vi "XML_method_params.vi"(0 "XML-message":string="<?xml version=\"1.0\"?>\n<methodCall>\n <methodName>jil.runvi</methodName>\n <params>\n   <param>\n     <value><i4>41</i4></value>\n   </param>\n   <param>\n     <value><int>-17</int></value>\n   </param>\n   <param>\n     <value><boolean>1</boolean></value>\n   </param>\n   <param>\n     <value><string>Hola</string></value>\n   </param>\n   <param>\n     <value>esto es un string \"a pelo\"</value>\n   </param>\n   <param>\n     <value><double>-187.217</double></value>\n   </param>\n   <param>\n     <value><dateTime.iso8601>19980717T14:08:55</dateTime.iso8601></value>\n   </param>\n   <param>\n     <value><base64>eW91IGNhbid0IHJlYWQgdGhpcyE=</base64></value>\n   </param>\n\n   <param>\n     <value>\n     <struct>\n       <member>\n            <name>lowerBound</name>\n           <value><i4>18</i4></value>\n       </member>\n        <member>\n           <name>upperBound</name>\n           <value><i4>139</i4></value>\n         </member>\n       </struct>\n      </value>\n   </param>\n\n   <param>\n     <value>\n     <array>\n        <data>\n           <value><i4>12</i4></value>\n           <value><string>Egypt</string></value>\n           <value><boolean>0</boolean></value>\n           <value><i4>-31</i4></value>\n        </data>\n       </array>\n      </value>\n    </param>\n\n </params>\n</methodCall>\n\n" caption="Result") -> (1 "ParsingErrors":string="<?xml version=\"1.0\" encoding=\"UTF-8\"?>\n<methodResponse>\n  <fault>\n    <value>\n      <struct>\n        <member>\n          <name>faultCode</name>\n          <value><int>811</int></value>\n        </member>\n        <member>\n          <name>faultString</name>\n          <value><string>Error in value:\n\" &ampvalue>\n     <value><i4>41</i4></value>\n   </value>\"</string></value>\n        </member>\n     </struct>\n    </value>\n  </fault>\n</methodResponse>", 2 "Values":variant[](array[variant]), 3 "Types":T1(array[ring])=[enum."int"], 4 "Method":T2(ring)=enum."RunVI")   [LabVIEW 2010]
panel:
  out "tag_list":string[](array[string])
  out "body_temp":string="\n\n"
  out "XML ok":bool
  out "RestOfParams":string
  out "XMLparams":string[](array[string])=["\n     <value><i4>41</i4></value>\n   ", "\n     <value><int>-17</int></value>\n   ", "\n     <value><boolean>1</boolean></value>\n   ", "\n     <value><string>Hola</string></value>\n   ", "\n     <value>esto es un string \"a pelo\"</value>\n   ", "\n     <value><double>-187.217</double></value>\n   ", "\n     <value><dateTime.iso8601>19980717T14:08:55</dateTime.iso8601></value>\n   ", "\n     <value><base64>eW91IGNhbid0IHJlYWQgdGhpcyE=</base64></value>\n   ", "\n     <value>\n     <struct>\n       <member>\n            <name>lowerBound</name>\n           <value><i4>18</i4></value>\n       </member>\n        <member>\n           <name>upperBound</name>\n           <value><i4>139</i4></value>\n         </member>\n       </struct>\n      </value>\n   ", "\n     <value>\n     <array>\n        <data>\n           <value><i4>12</i4></value>\n           <value><string>Egypt</string></value>\n           <value><boolean>0</boolean></value>\n           <value><i4>-31</i4></value>\n        </data>\n       </array>\n      </value>\n    "]
  out "header":string="<?xml version=\"1.0\"?>"
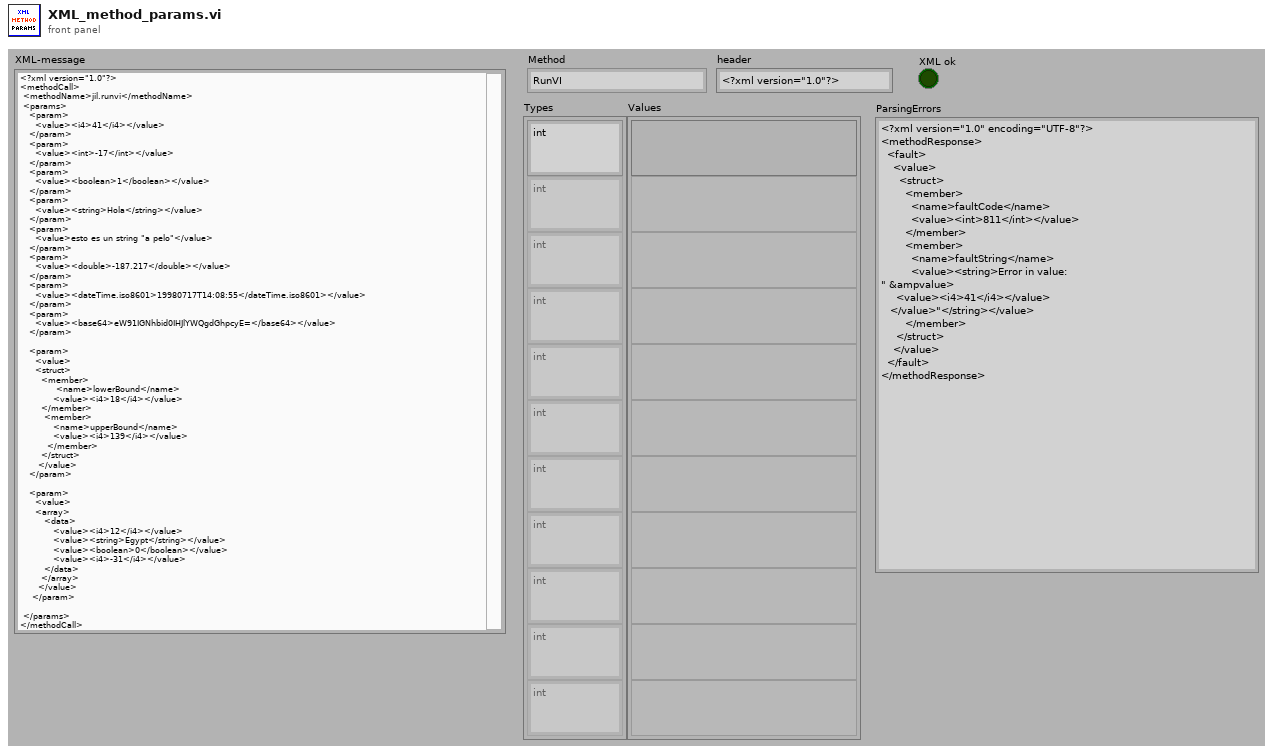
[diagram p1: front panel]
types:
  T1 = enum16{"int", "boolean", "string", "double", "dateTime", "base64", "struct", "array"}[]
  T2 = enum16{"Connect", "Authenticate", "OpenVI", "RunVI", "SyncVI", "StopVI", "CloseVI", "Disconnect"}
  T3 = enum16{"int", "boolean", "string", "double", "dateTime", "base64", "struct", "array"}
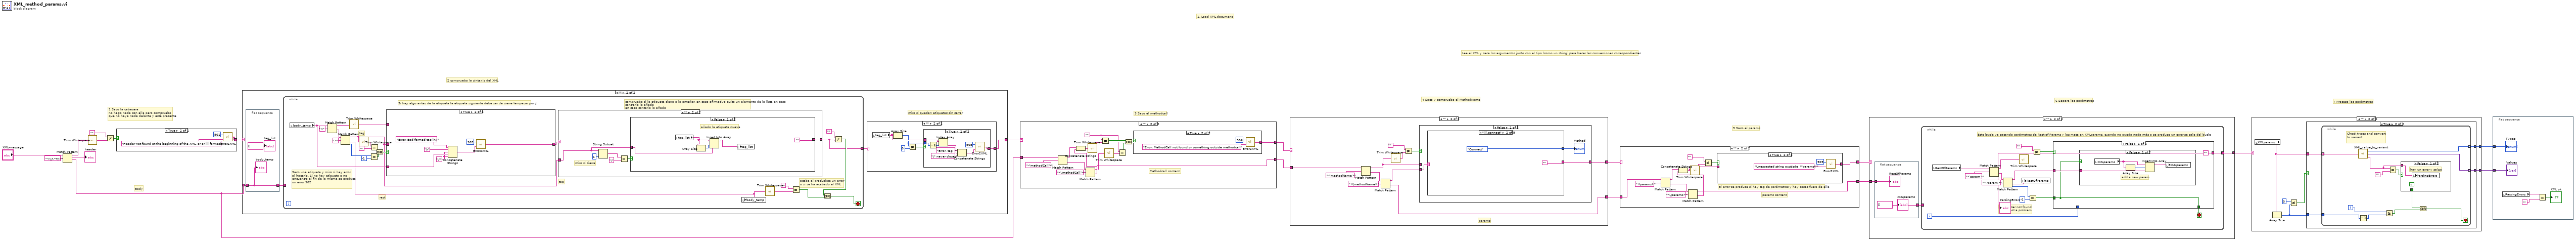
[diagram p0: block diagram]
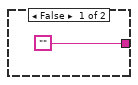
[diagram p2: hidden frame]
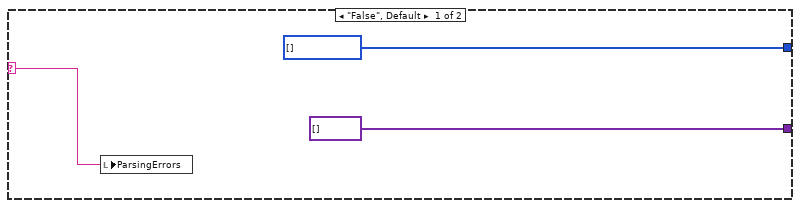
[diagram p3: hidden frame]
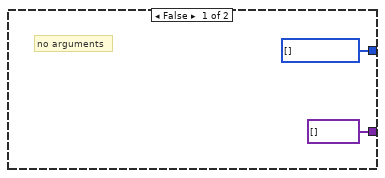
[diagram p4: hidden frame]
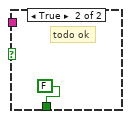
[diagram p5: hidden frame]
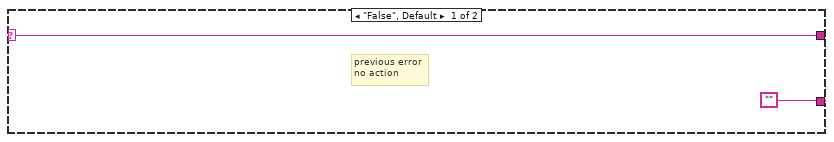
[diagram p6: hidden frame]
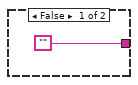
[diagram p7: hidden frame]
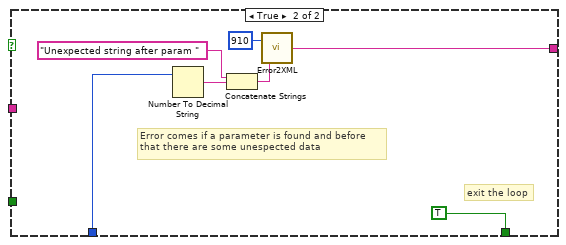
[diagram p10: hidden frame]
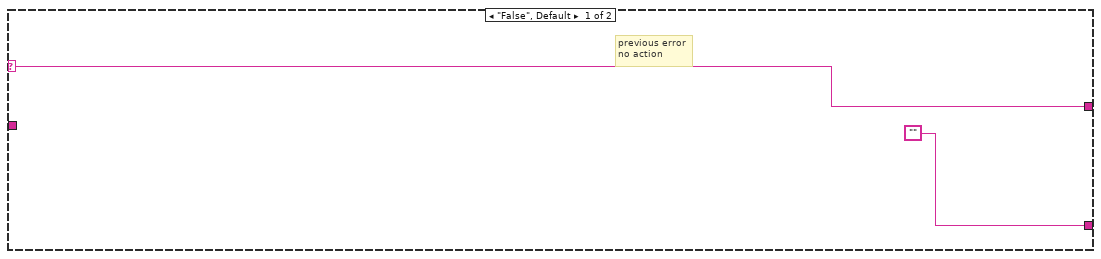
[diagram p11: hidden frame]
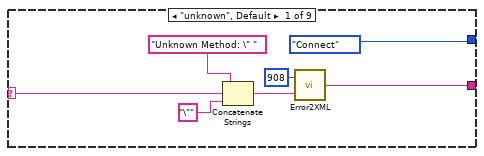
[diagram p12: hidden frame]
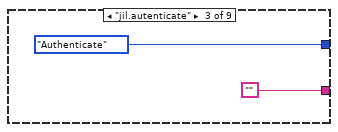
[diagram p13: hidden frame]
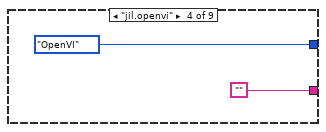
[diagram p14: hidden frame]
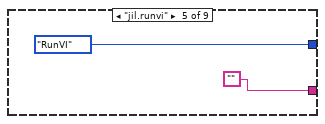
[diagram p15: hidden frame]
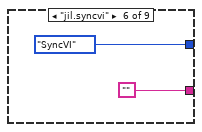
[diagram p16: hidden frame]
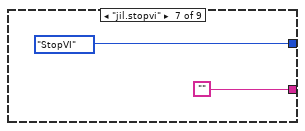
[diagram p17: hidden frame]
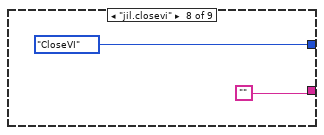
[diagram p18: hidden frame]
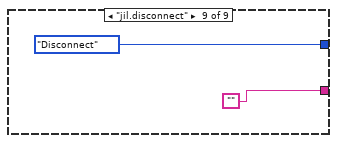
[diagram p19: hidden frame]
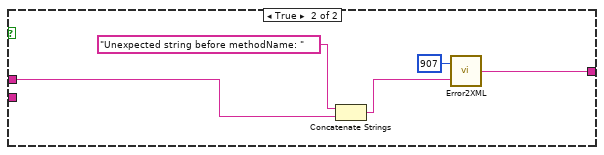
[diagram p20: hidden frame]
diagram:
  # "7 Proceso los parámetros"
  # "6 Separa los parámetros"
  # "5 Saco el params"
  # "4 Saco y compruebo el MethodName"
  # "3 Saco el methodcall"
  # "1 Saco la cabecera\nno hago nada con ella pero compruebo \nque no haya nada delante y esté presente"
  # "Body"
  # "2 compruebo la sintaxis del XML"
  # "1. Load XML document"
  # "Lee el XML y saca los argumentos junto con el tipo (como un string) para hacer las conversiones correspondientes"
  n1 = Match Pattern(string="XML-message", regular expression="<\\?.*?\\>") -> (before substring=w8:string, match substring=→"header":string, after substring=w2:string)  [unwired: 1 in, 1 out]
  n2 = call <vilib>:"Trim Whitespace.vi"("string"=w8) -> ("trimmed string"=w9:string)  [unwired: 1 in]
  n3 = Not Equal?(x="", y=w9) -> (x != y?=w5:bool)
  n4 = case shown="True" w5 {
    tunnel: ["" w21] -> w3
    frame False {
    }
    frame True {
      n5 = call "Error2XML.vi"("FailDescriptor"="Header not found at the beginning of the XML, or or ill formed ", "FailID"=901) -> ("ErrorXML"=w21:string)
    }
  }
  n6 = case shown="\"\"" w3 {
    selector: w3 -> [w24 _]
    tunnel: [w24 w25] -> w19
    tunnel: w2 -> [_ w28]
    frame "False", Default {
      # "previous error\nno action"
    }
    frame "" {
      # "miro si quedan etiquetas sin cerrar"
      n7 = flat-sequence {
        tunnel: [w46] -> w27
        tunnel: w28 -> [w46]
        frame #0 {
          "body_temp" <- w46
          "tag_list" <- string[] [] ("tag_list")
        }
      }
      n8 = while {
        tunnel: w27 -> [_]
        tunnel: [w52] -> w26
        stop <- w53 stop-if-true
        # "rest"
        # "tag"
        # "acaba al producirse un error\no si se ha acabado el XML"
        # "tag"
        # "Saco una etiqueta y miro si hay error\nal hacerlo. Si no hay etiqueta o no encuentro el fin de la misma se produce un error 902"
        # "compruebo si la etiqueta cierra a la anterior, en caso afirmativo quito un elemento de la lista en caso contrario lo añado\nen caso contario lo añado"
        # "Si hay algo antes de la etiqueta la etiqueta siguiente debe ser de cierre (empezar por /)"
        n9 = local read "body_temp"() -> (w49:string)
        n10 = Match Pattern(string=w49, regular expression="<") -> (before substring=w50:string, after substring=w68:string)  [unwired: 1 in, 2 out]
        n11 = Match Pattern(string=w68, regular expression=">") -> (before substring=w51:string, after substring=w47:string, offset past match=w58:i32)  [unwired: 1 in, 1 out]
        n12 = call <vilib>:"Trim Whitespace.vi"("string"=w50) -> ("trimmed string"=w66:string)  [unwired: 1 in]
        n13 = call <vilib>:"Trim Whitespace.vi"("string"=w51) -> ("trimmed string"=w59:string)  [unwired: 1 in]
        n14 = Equal?(x=w58, y=-1) -> (x = y?=w54:bool)
        n15 = Equal?(x=w59, y="") -> (x = y?=w55:bool)
        n16 = Or(x=w55, y=w54) -> (x .or. y?=w56:bool)
        n17 = case shown="True" w56 {
          tunnel: w66 -> [w72 _]
          tunnel: [w71 w91] -> w65
          tunnel: w51 -> [w70 _]
          tunnel: w49 -> [_ w88]
          frame False {
            n18 = case shown="\"False\", Default" w72 {
              selector: w72 -> [w74 _]
              tunnel: [w75 ""] -> w71
              tunnel: w70 -> [w73 _]
              frame "False", Default {
                n19 = String Subset(string=w73, length (rest)=1 ("length (rest)")) -> (substring=w78:string)  [unwired: 1 in]
                n20 = Not Equal?(x=w78, y="/") -> (x != y?=w76:bool)
                n21 = case shown="True" w76 {
                  tunnel: w74 -> [_ w84]
                  tunnel: ["" w81] -> w75
                  frame False {
                  }
                  frame True {
                    n22 = Concatenate Strings("Text not enclosed into tags: ", w84) -> (w82:string)
                    n23 = call "Error2XML.vi"("FailDescriptor"=w82, "FailID"=903) -> ("ErrorXML"=w81:string)
                  }
                }
              }
              frame "" {
              }
            }
          }
          frame True {
            w87 = "\"" ("string")
            n24 = Concatenate Strings("Error: Bad formed tag in: " ("string"), "\r", w87, w88, w87) -> (w92:string)
            n25 = call "Error2XML.vi"("FailDescriptor"=w92, "FailID"=902) -> ("ErrorXML"=w91:string)
          }
        }
        n26 = case shown="\"\"" w65 {
          selector: w65 -> [w94 _]
          tunnel: [w94 w95] -> w52
          tunnel: w51 -> [_ w96]
          frame "False", Default {
          }
          frame "" {
            # "miro si cierra"
            n27 = String Subset(string=w96, length (rest)=1 ("length (rest)")) -> (substring=w99:string)  [unwired: 1 in]
            n28 = Equal?(x=w99, y="/") -> (x = y?=w97:bool)
            n29 = case shown="False" w97 {
              tunnel: w96 -> [w101 w107]
              tunnel: ["" w106] -> w95
              frame False {
                # "añado la etiqueta nueva"
                n30 = local read "tag_list"() -> (w103:string[])
                n31 = Array Size(array=w103) -> (size(s)=w102:i32)
                n32 = Insert Into Array(array=w103, index=w102, new element=w101) -> (w104:string[])
                n33 = local write "tag_list"(w104) -> ()
              }
              frame True {
                # "etiqueta anterior"
                # "Debería cerrar a la etiqueta anterior"
                n34 = local read "tag_list"() -> (w114:string[])
                n35 = Array Size(array=w114) -> (size(s)=w113:i32)
                n36 = Decrement(x=w113) -> (x-1=w109:i32)
                n37 = Index Array(array=w114, index=w109) -> (element=w108:string)
                n38 = Concatenate Strings("/" ("string"), w108) -> (w111:string)
                n39 = Equal?(x=w111, y=w107) -> (x = y?=w110:bool)
                n40 = case shown="True" w110 {
                  tunnel: w109 -> [_ w124]
                  tunnel: w108 -> [w121 _]
                  tunnel: w107 -> [w118 _]
                  tunnel: [w115 ""] -> w106
                  frame False {
                    n41 = Concatenate Strings("Error: trying to close \" " ("FailDescriptor"), w121, "\" with \"" ("string"), w118, "\"") -> (w116:string)
                    n42 = call "Error2XML.vi"("FailDescriptor"=w116, "FailID"=904) -> ("ErrorXML"=w115:string)
                  }
                  frame True {
                    # "quito la etiqueta anterior"
                    n43 = local read "tag_list"() -> (w126:string[])
                    n44 = Delete From Array(array=w126, length=1, index=w124) -> (array with subset deleted=w127:string[])  [unwired: 1 out]
                    n45 = local write "tag_list"(w127) -> ()
                  }
                }
              }
            }
          }
        }
        n46 = local write "body_temp"(w47) -> ()
        n47 = call <vilib>:"Trim Whitespace.vi"("string"=w47) -> ("trimmed string"=w48:string)  [unwired: 1 in]
        n48 = Equal?(x="", y=w48) -> (x = y?=w63:bool)
        n49 = Not Equal?(x="", y=w52) -> (x != y?=w61:bool)
        n50 = Or(x=w61, y=w63) -> (x .or. y?=w53:bool)
      }
      n51 = case shown="\"\"" w26 {
        selector: w26 -> [w29 _]
        tunnel: [w29 w30] -> w25
        frame "False", Default {
        }
        frame "" {
          n52 = local read "tag_list"() -> (w32:string[])
          n53 = Array Size(array=w32) -> (size(s)=w31:i32)
          n54 = Not Equal?(x=w31, y=0) -> (x != y?=w33:bool)
          n55 = case shown="True" w33 {
            tunnel: w32 -> [_ w42]
            tunnel: w31 -> [_ w44]
            tunnel: ["" w36] -> w30
            frame False {
            }
            frame True {
              n56 = Decrement(x=w44) -> (x-1=w43:i32)
              n57 = Index Array(array=w42, index=w43) -> (element=w40:string)
              n58 = Concatenate Strings("Error, tag “" ("string"), w40, "\" never closed" ("string")) -> (w38:string)
              n59 = call "Error2XML.vi"("FailDescriptor"=w38, "FailID"=905) -> ("ErrorXML"=w36:string)
            }
          }
        }
      }
    }
  }
  n60 = case shown="\"\"" w19 {
    selector: w19 -> [w129 _]
    tunnel: w2 -> [_ w143]
    tunnel: ["" w130] -> w18
    tunnel: [w129 w142] -> w17
    frame "False", Default {
      # "previous error\nno action"
    }
    frame "" {
      w135 = ""
      # "Methodcall content"
      n61 = Match Pattern(string=w143, regular expression="<methodCall>") -> (before substring=w141:string, after substring=w132:string)  [unwired: 1 in, 2 out]
      n62 = Match Pattern(string=w132, regular expression="</methodCall>") -> (before substring=w130:string, after substring=w131:string)  [unwired: 1 in, 2 out]
      n63 = Concatenate Strings(w141, w131) -> (w140:string)
      n64 = call <vilib>:"Trim Whitespace.vi"("string"=w140) -> ("trimmed string"=w139:string)  [unwired: 1 in]
      n65 = Not Equal?(x=w135, y=w139) -> (x != y?=w137:bool)
      n66 = call <vilib>:"Trim Whitespace.vi"("string"=w130) -> ("trimmed string"=w136:string)  [unwired: 1 in]
      n67 = Equal?(x=w135, y=w136) -> (x = y?=w134:bool)
      n68 = Or(x=w137, y=w134) -> (x .or. y?=w138:bool)
      n69 = case shown="True" w138 {
        tunnel: ["" w146] -> w142
        frame False {
        }
        frame True {
          n70 = call "Error2XML.vi"("FailDescriptor"="Error: MethodCall not found or something outside methodcall", "FailID"=906) -> ("ErrorXML"=w146:string)
        }
      }
    }
  }
  n71 = case shown="\"\"" w17 {
    selector: w17 -> [w150 _]
    tunnel: w18 -> [_ w160]
    tunnel: ["" w152] -> w1
    tunnel: [w150 w159] -> w16
    frame "False", Default {
      # "previous error\nno action"
    }
    frame "" {
      # "params"
      n72 = Match Pattern(string=w160, regular expression="<methodName>") -> (before substring=w151:string, after substring=w153:string)  [unwired: 1 in, 2 out]
      n73 = Match Pattern(string=w153, regular expression="</methodName>") -> (before substring=w154:string, after substring=w152:string)  [unwired: 1 in, 2 out]
      n74 = call <vilib>:"Trim Whitespace.vi"("string"=w151) -> ("trimmed string"=w156:string)  [unwired: 1 in]
      n75 = Not Equal?(x="", y=w156) -> (x != y?=w157:bool)
      n76 = case shown="False" w157 {
        tunnel: [w164 w191] -> w159
        tunnel: w154 -> [w163 _]
        tunnel: w151 -> [_ w190]
        frame False {
          n77 = case shown="\"jil.connect\"" w163 {
            selector: w163 -> [w166 _ _ _ _ _ _ _ _]
            tunnel: [w167 "" "" "" "" "" "" "" ""] -> w164
            tunnel: [T2."Connect" ("Method") T2."Connect" ("Method") T2."Authenticate" ("Method") T2."OpenVI" ("Method") T2."RunVI" ("Method") T2."SyncVI" ("Method") T2."StopVI" ("Method") T2."CloseVI" ("Method") T2."Disconnect" ("Method")] -> w162
            frame "unknown", Default {
              n78 = Concatenate Strings("Unknown Method: \" " ("FailDescriptor"), w166, "\"" ("string")) -> (w169:string)
              n79 = call "Error2XML.vi"("FailDescriptor"=w169, "FailID"=908) -> ("ErrorXML"=w167:string)
            }
            frame "jil.connect" {
            }
            frame "jil.autenticate" {
            }
            frame "jil.openvi" {
            }
            frame "jil.runvi" {
            }
            frame "jil.syncvi" {
            }
            frame "jil.stopvi" {
            }
            frame "jil.closevi" {
            }
            frame "jil.disconnect" {
            }
          }
          "Method" <- w162
        }
        frame True {
          n80 = Concatenate Strings("Unexpected string before methodName: " ("FailDescriptor"), w190) -> (w188:string)
          n81 = call "Error2XML.vi"("FailDescriptor"=w188, "FailID"=907) -> ("ErrorXML"=w191:string)
        }
      }
    }
  }
  n82 = case shown="\"\"" w16 {
    selector: w16 -> [w194 _]
    tunnel: w1 -> [_ w205]
    tunnel: ["" w198] -> w14
    tunnel: [w194 w204] -> w15
    frame "False", Default {
      # "previous error\nno action"
    }
    frame "" {
      # "El error se produce si hay tag de parámetros y hay cosas fuera de ella"
      # "params content"
      n83 = Match Pattern(string=w205, regular expression="<params>") -> (before substring=w203:string, after substring=w200:string)  [unwired: 1 in, 2 out]
      n84 = Match Pattern(string=w200, regular expression="</params>") -> (before substring=w198:string, after substring=w199:string)  [unwired: 1 in, 2 out]
      n85 = Concatenate Strings(w203, w199) -> (w195:string)
      n86 = call <vilib>:"Trim Whitespace.vi"("string"=w195) -> ("trimmed string"=w202:string)  [unwired: 1 in]
      n87 = Not Equal?(x="", y=w202) -> (x != y?=w196:bool)
      n88 = case shown="True" w196 {
        tunnel: ["" w208] -> w204
        tunnel: w195 -> [_ _]
        frame False {
        }
        frame True {
          n89 = call "Error2XML.vi"("FailDescriptor"="Unespected string oustisde  \"params\"", "FailID"=909) -> ("ErrorXML"=w208:string)
        }
      }
    }
  }
  n90 = case shown="\"\"" w15 {
    selector: w15 -> [w211 _]
    tunnel: w14 -> [_ w213]
    tunnel: [w211 w214] -> w13
    frame "False", Default {
      # "previous error\nno action"
    }
    frame "" {
      n91 = flat-sequence {
        tunnel: w213 -> [w216]
        tunnel: [w215] -> w212
        frame #0 {
          w215 = string[] [] ("XMLparams")
          "XMLparams" <- w215
          "RestOfParams" <- w216
        }
      }
      n92 = while {
        tunnel: [w226] -> w214
        tunnel: w212 -> [_]
        i -> [w227]
        stop <- w223 stop-if-true
        # "Este bucle va sacando parámetros de Rest of Params y los mete en XMLparams, cuando no queda nada más o se produce un error se sale del bucle"
        # "parameter not found\nthis is not a problem"
        n93 = local read "RestOfParams"() -> (w219:string)
        n94 = Match Pattern(string=w219, regular expression="<param>") -> (before substring=w230:string, after substring=w221:string)  [unwired: 1 in, 2 out]
        n95 = Match Pattern(string=w221, regular expression="</param>") -> (before substring=w217:string, after substring=w218:string, offset past match=w220:i32)  [unwired: 1 in, 1 out]
        n96 = call <vilib>:"Trim Whitespace.vi"("string"=w230) -> ("trimmed string"=w229:string)  [unwired: 1 in]
        n97 = local write "RestOfParams"(w218) -> ()
        n98 = Equal?(x=w220, y=-1) -> (x = y?=w224:bool)
        n99 = Not Equal?(x="", y=w229) -> (x != y?=w228:bool)
        n100 = case shown="False" w228 {
          tunnel: w227 -> [_ w245]
          tunnel: ["" w242] -> w226
          tunnel: w224 -> [w233 _]
          tunnel: w217 -> [w234 _]
          tunnel: [w233 TRUE] -> w223
          frame False {
            n101 = case shown="False" w233 {
              tunnel: w234 -> [w238 _]
              frame False {
                # "add a new param"
                n102 = local read "XMLparams"() -> (w239:string[])
                n103 = Array Size(array=w239) -> (size(s)=w236:i32)
                n104 = Insert Into Array(array=w239, index=w236, new element=w238) -> (w237:string[])
                n105 = local write "XMLparams"(w237) -> ()
              }
              frame True {
              }
            }
          }
          frame True {
            # "Error comes if a parameter is found and before\nthat there are some unespected data"
            # "exit the loop"
            n106 = Number To Decimal String(number=w245) -> (decimal integer string=w244:string)  [unwired: 1 in]
            n107 = Concatenate Strings("Unexpected string after param " ("FailDescriptor"), w244) -> (w240:string)
            n108 = call "Error2XML.vi"("FailDescriptor"=w240, "FailID"=910) -> ("ErrorXML"=w242:string)
          }
        }
      }
    }
  }
  "ParsingErrors" <- w13
  n109 = case shown="\"\"" w13 {
    selector: w13 -> [w247 _]
    tunnel: [w249 w255] -> w12
    tunnel: [variant[] [] w254] -> w11
    frame "False", Default {
      w249 = T1 [] items=["int", "boolean", "string", "double", "dateTime", "base64", "struct", "array"]
      n110 = local write "ParsingErrors"(w247) -> ()
    }
    frame "" {
      n111 = local read "XMLparams"() -> (w253:string[])
      n112 = Array Size(array=w253) -> (size(s)=w252:i32)
      n113 = Not Equal?(x=0, y=w252) -> (x != y?=w250:bool)
      n114 = case shown="True" w250 {
        tunnel: [w257 w261] -> w255
        tunnel: [variant[] [] w260] -> w254
        tunnel: w253 -> [_ w259]
        tunnel: w252 -> [_ w258]
        frame False {
          w257 = T1 [] items=["int", "boolean", "string", "double", "dateTime", "base64", "struct", "array"]
          # "no arguments"
        }
        frame True {
          n115 = while {
            tunnel: w259 -> [w262] mode=indexing
            tunnel: [w273] -> w261 mode=indexing
            tunnel: [w272] -> w260 mode=indexing
            tunnel: w258 -> [w263]
            i -> [w265]
            stop <- w266 stop-if-true
            # "Check types and convert\nto variant"
            n116 = call "XML_value_to_variant.vi"("XML-param"=w262) -> ("ParsingErrors"=w267:string, "Value"=w272:variant, "Type"=w273:T3)
            n117 = Decrement(x=w263) -> (x-1=w264:i32)
            n118 = Greater Or Equal?(x=w265, y=w264) -> (x >= y?=w271:bool)
            n119 = Equal?(x=w267, y="") -> (x = y?=w269:bool)
            n120 = case shown="False" w269 {
              tunnel: [TRUE FALSE] -> w268
              tunnel: w267 -> [w275 _]
              frame False {
                # "hay un error y salgo"
                n121 = local write "ParsingErrors"(w275) -> ()
              }
              frame True {
                # "todo ok"
              }
            }
            n122 = Or(x=w268, y=w271) -> (x .or. y?=w266:bool)
          }
        }
      }
    }
  }
  n123 = flat-sequence {
    tunnel: w12 -> [w278]
    tunnel: w11 -> [w277]
    frame #0 {
      n124 = local read "ParsingErrors"() -> (w281:string)
      n125 = Equal?(x=w281, y="") -> (x = y?=→"XML ok":bool)
      "Types" <- w278
      "Values" <- w277
    }
  }
